vi "Set VI Description.vi"(8 "error in (no error)":errorcluster, 10 "VI Description":string, 11 "VI":refnum<vi>) -> (0 "error out":errorcluster, 3 "VI out":refnum<vi>)   [LabVIEW 2014]
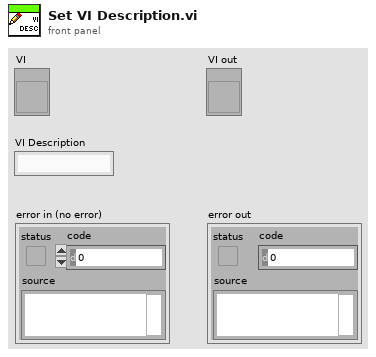
[diagram p1: front panel]
types:
  T1 = typedef "TYPE_Description Cluster.ctl" = cluster{"VI Description":string, "VI Version":string, "Review Date":string, "Author":string, "Copyright":string, "Requirements Coverage":string}
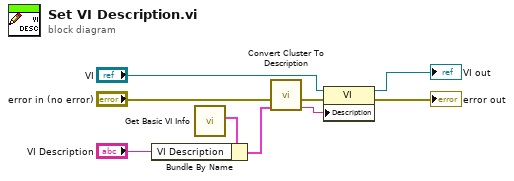
[diagram p0: block diagram]
diagram:
  n1 = call "Get Basic VI Info.vi"() -> ("VI Description Info"=w9:T1)  [unwired: 11 in]
  n2 = Bundle By Name(cluster=w9, "VI Description"="VI Description") -> (w7:T1)
  n3 = call "Convert Cluster To Description.vi"("Description Cluster"=w7, "error in (no error)"="error in (no error)") -> ("Description String (empty)"=w5:string, "error out"=w4:errorcluster)  [unwired: 8 in]
  n4 = property class="VI"(reference="VI", error in=w4, "Description"=w5) -> (reference out=→"VI out":refnum<vi>, error out=→"error out":errorcluster)
